vi "GetCountRates.vi"(3 "error in (no error)":errorcluster, 5 "DeviceIndex":i32) -> (0 "error out":errorcluster, 1 "CntRates":dbl[](array[numeric]), 2 "SyncRate":i32)   [LabVIEW 2013]
uses:
  MT Scan/SubVIs/hhlib.dll
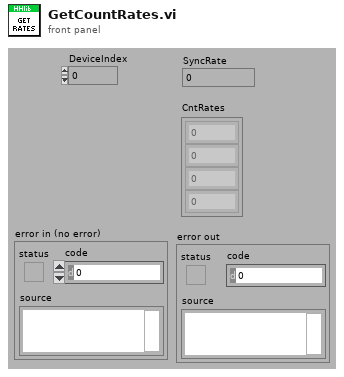
[diagram p1: front panel]
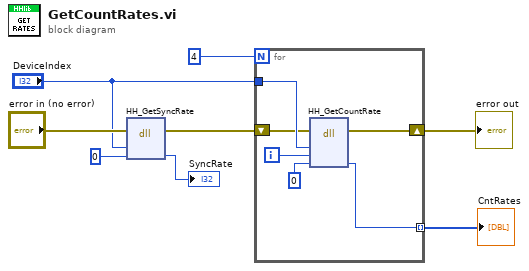
[diagram p0: block diagram]
diagram:
  n1 = dll-call lib="C:/Documents and Settings/PQ/My Documents/Eigene VIs/MTSetupNew/MT Scan/SubVIs/hhlib.dll" fn="HH_GetSyncRate"(error in="error in (no error)", "devidx"="DeviceIndex", "rate"=0) -> (error out=w4:errorcluster, "rate"=→"SyncRate":i32)  [unwired: 4 in, 1 out]
  n2 = for {
    N: 4 -> [_]
    tunnel: "DeviceIndex" -> [w12]
    shift-right: [w10] -> w3
    shift-left: w4 -> [w11]
    tunnel: [w9] -> w2 mode=indexing
    i -> [w13]
    n3 = dll-call lib="C:/Documents and Settings/PQ/My Documents/Eigene VIs/MTSetupNew/MT Scan/SubVIs/hhlib.dll" fn="HH_GetCountRate"(error in=w11, "devidx"=w12, "channel"=w13, "rate"=0) -> (error out=w10:errorcluster, "rate"=w9:i32)  [unwired: 5 in, 1 out]
  }
  "error out" <- w3
  "CntRates" <- w2
